vi "ComputeFlowrates.vi"(4 "minFlowrate (l/min)":dbl min=0.0 max=360.0 step=1.0 format="%.2f", 5 "Pressure channel":string, 6 "maxFlowrate (l/min)":dbl min=0.0 max=360.0 step=1.0 format="%.2f", 7 "Temperature channel":string, 9 "C_dem:(%)":dbl, 10 "Q_dem[Total]:(l/min)":dbl, 11 "DataBus in":T1 {"RhoTrace" format="%.3gg/l"; "RhoCarrier" format="%.3gg/l"; "InactiveC2H6MFCs"."Setpoint" format="%_4g"; "ActiveC2H6MFCs"."Setpoint" format="%_4g"; "InactiveN2MFCs"."Setpoint" format="%_4g"; "ActiveN2MFCs"."Setpoint" format="%_4g"; "C2H6MFCs"."Setpoint" format="%_4g"; "N2MFCs"."Setpoint" format="%_4g"; "QdemCarrier" format="%.2pl/min"; "QdemTrace" format="%.2pl/min"; "MdotCarrier" format="%_4pg/min"; "MdotTrace" format="%_4pg/min"; "Temp" format="%#_gC"; "Press" format="%#_gmBar"}) -> (3 "DataBus out":T1 {"RhoTrace" format="%.3gg/l"; "RhoCarrier" format="%.3gg/l"; "InactiveC2H6MFCs"."Setpoint" format="%_4g"; "ActiveC2H6MFCs"."Setpoint" format="%_4g"; "InactiveN2MFCs"."Setpoint" format="%_4g"; "ActiveN2MFCs"."Setpoint" format="%_4g"; "C2H6MFCs"."Setpoint" format="%_4g"; "N2MFCs"."Setpoint" format="%_4g"; "QdemCarrier" format="%.2pl/min"; "QdemTrace" format="%.2pl/min"; "MdotCarrier" format="%_4pg/min"; "MdotTrace" format="%_4pg/min"; "Temp" format="%#_gC"; "Press" format="%#_gmBar"})   [LabVIEW 2016]
uses:
  AalborgServerData.ctl
  MFCdescription.ctl
  MFCcapability.ctl
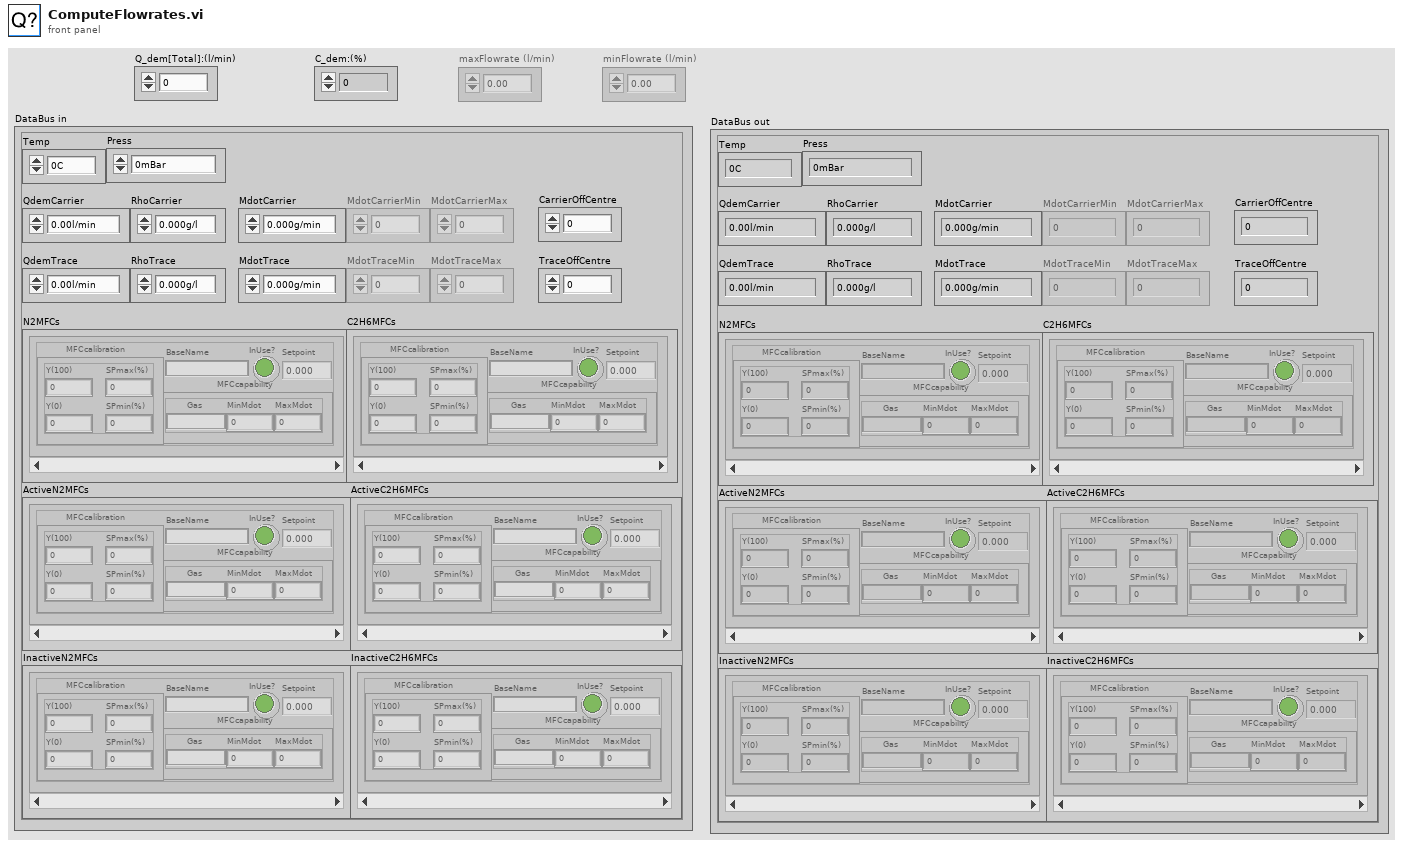
[diagram p1: front panel]
types:
  T1 = typedef "AalborgServerData.ctl" = cluster{"Temp":dbl, "Press":dbl, "QdemCarrier":dbl, "QdemTrace":dbl, "MdotCarrier":dbl, "MdotCarrierMin":dbl, "MdotCarrierMax":dbl, "MdotTrace":dbl, "MdotTraceMin":dbl, "MdotTraceMax":dbl, "N2MFCs":T2[], "C2H6MFCs":T2[], "CarrierOffCentre":dbl, "TraceOffCentre":dbl, "ActiveN2MFCs":T2[], "InactiveN2MFCs":T2[], "ActiveC2H6MFCs":T2[], "InactiveC2H6MFCs":T2[], "RhoCarrier":dbl, "RhoTrace":dbl}
  T2 = typedef "MFCdescription.ctl" = cluster{"BaseName":string, "MFCcalibration":cluster{"Y(100)":dbl, "Y(0)":dbl, "SPmin(%)":dbl, "SPmax(%)":dbl}, "MFCcapability":T3, "InUse?":bool, "Setpoint":dbl}
  T3 = typedef "MFCcapability.ctl" = cluster{"Gas":string, "MinMdot":dbl, "MaxMdot":dbl}
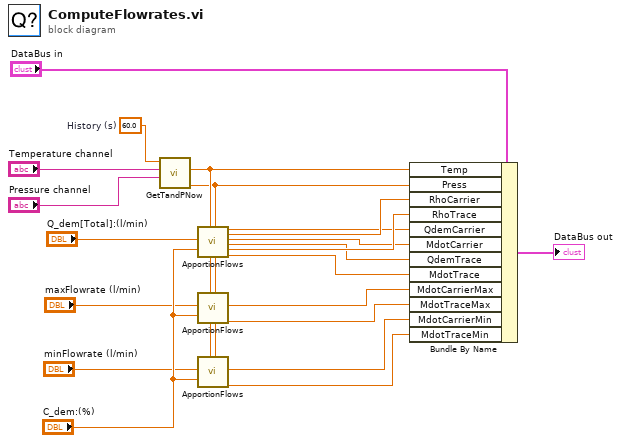
[diagram p0: block diagram]
diagram:
  w17 = 60.0  # History (s)
  n1 = call "GetTandPNow.vi"("Pressure channel"="Pressure channel", "Temperature channel"="Temperature channel", "History (s)"=w17) -> ("Press (mBar)"=w1:dbl, "Temp (C)"=w15:dbl)  [unwired: 7 in]
  n2 = call "ApportionFlows.vi"("Q[Total]:(l/min)"="Q_dem[Total]:(l/min)", "C:(%)"="C_dem:(%)", "Temp (C)"=w15, "Press (mBar)"=w1) -> ("Q[N2]:(l/min)"=w9:dbl, "Rho[N2]:(kg/l)"=w11:dbl, "Mdot[N2]:(g/min)"=w8:dbl, "Q[Ethane]:(l/min)"=w7:dbl, "Rho[Ethane]:(kg/l)"=w10:dbl, "Mdot[Ethane]:(g/min)"=w6:dbl)  [unwired: 10 in]
  n3 = call "ApportionFlows.vi"("Q[Total]:(l/min)"="maxFlowrate (l/min)", "C:(%)"="C_dem:(%)", "Temp (C)"=w15, "Press (mBar)"=w1) -> ("Mdot[N2]:(g/min)"=w5:dbl, "Mdot[Ethane]:(g/min)"=w4:dbl)  [unwired: 10 in, 4 out]
  n4 = call "ApportionFlows.vi"("Q[Total]:(l/min)"="minFlowrate (l/min)", "C:(%)"="C_dem:(%)", "Temp (C)"=w15, "Press (mBar)"=w1) -> ("Mdot[N2]:(g/min)"=w3:dbl, "Mdot[Ethane]:(g/min)"=w2:dbl)  [unwired: 10 in, 4 out]
  n5 = Bundle By Name(cluster="DataBus in", "Temp"=w15, "Press"=w1, "RhoCarrier"=w11, "RhoTrace"=w10, "QdemCarrier"=w9, "MdotCarrier"=w8, "QdemTrace"=w7, "MdotTrace"=w6, "MdotCarrierMax"=w5, "MdotTraceMax"=w4, "MdotCarrierMin"=w3, "MdotTraceMin"=w2) -> (→"DataBus out":T1)
